vi "Mod_OFDM_Examine_Configure_Modulator_Sources.vi"(0 "Configuration in":variant, 11 "error in":errorcluster) -> (4 "Configuration out":variant, 15 "error out":errorcluster)   [LabVIEW 2010]
doc: "The VI performs three functions:\n\n1) Examine pool of modulator sources that have been configured.\n\n2) Add/Edit the current pool of modulators. By default four Modulators are pre-configured.\n\n3) To store the current pool of modulators in the configuration Variant"
uses:
  Polymorphic_Sub_VI's/Mod_OFDM_Get_Modulator_Sources.vi
  Polymorphic_Sub_VI's/Mod_OFDM_Set_Modulator_Source.vi
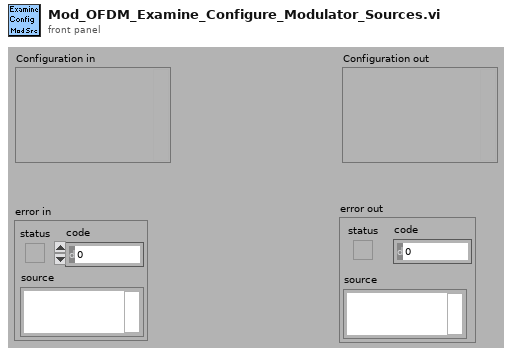
[diagram p1: front panel]
types:
  T1 = typedef "Pool of Modulator Control.ctl" = cluster{"M-QAM":enum16{"4", "16", "64", "256"}, "M-PSK":enum16{"2", "4", "8", "16", "32", "64", "128", "256"}, "Type of Modulation":enum16{"PSK", "QAM"}, " PSK":cluster{"differential PSK":enum16{"disable", "enable"}, "PSK type":enum16{"normal", "shifted", "offset"}}}[]
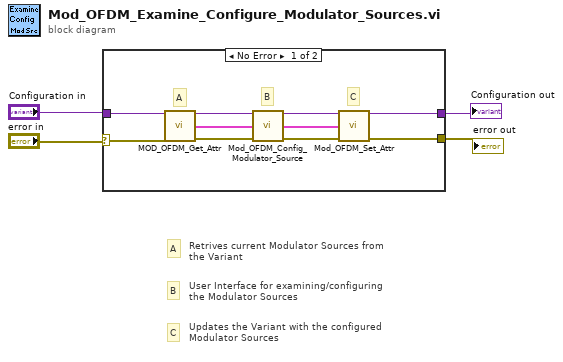
[diagram p0: block diagram]
diagram:
  # "Updates the Variant with the configured Modulator Sources"
  # "User Interface for examining/configuring the Modulator Sources"
  # "Retrives current Modulator Sources from the Variant"
  # "A"
  # "C"
  # "B"
  n1 = case shown="No Error" "error in" {
    selector: "error in" -> [w9 w15]
    tunnel: [w12 _] -> w4
    tunnel: "Configuration in" -> [w11 _]
    tunnel: [w10 w15] -> w2
    frame No Error {
      # "C"
      # "B"
      # "A"
      n2 = call-poly "MOD_OFDM_Get_Attr.vi"("Configuration in"=w11, "error in"=w9) -> ("Configuration out"=w8:variant, "Pool of Modulators"=w6:T1, "error out"=w14:errorcluster)  [unwired: 8 in, 3 out]
      n3 = call "Mod_OFDM_Config_Modulator_Source.vi"("Configuration in"=w8, "Pool of Modulators"=w6, "error in"=w14) -> ("Configuration out"=w7:variant, "Pool of Modulators"=w5:T1, "error out"=w13:errorcluster)  [unwired: 10 in]
      n4 = call-poly "Mod_OFDM_Set_Attr.vi"("Configuration in"=w7, "Pool of Modulators"=w5, "error in"=w13) -> ("Configuration out"=w12:variant, "error out"=w10:errorcluster)  [unwired: 11 in]
    }
    frame Error {
    }
  }
  "Configuration out" <- w4
  "error out" <- w2
